vi "Durability_will_2012_07_02_one thing.vi"() -> ()   [LabVIEW 2011]
uses:
  <vilib>/DAQmx/write.llb/DAQmx Write (Counter Time 1Chan 1Samp).vi
  <vilib>/DAQmx/read.llb/DAQmx Read (Analog 1D Wfm NChan NSamp).vi
  <vilib>/DAQmx/create/channels.llb/DAQmx Create Channel (CO-Pulse Generation-Time).vi
  <vilib>/DAQmx/configure/timing.llb/DAQmx Timing (Implicit).vi
  <vilib>/DAQmx/configure/timing.llb/DAQmx Timing (Sample Clock).vi
  <vilib>/DAQmx/create/channels.llb/DAQmx Create Channel (AI-Voltage-Basic).vi
  <vilib>/measure/madcrms.llb/Averaged DC-RMS for 1 Chan.vi
  <vilib>/DAQmx/miscellaneous.llb/DAQmx Fill In Error Info.vi
  <vilib>/measure/NI_MAPro.lvlib
  C:/Program Files/National Instruments/LabVIEW 2011/resource/objmgr/daqmx.rc
panel:
  in  "task in":refnum<k21>
  in  "Physical Channels":tag[](array[tag])
  in  "Channels Name":string[](array[string])
  out "VDE":waveform(dbl)
  out "ICD":waveform(dbl)
  out "VBE":waveform(dbl)
  out "IAB":waveform(dbl)
  out "RPM Graph":dbl(graph)
  out "Motor RPM":dbl format="%#.0f"
  out "Motor Power (watts)":dbl format="%#.4f"
  out "Motor Power Over Time":waveform(dbl)(graph)
  out "Phase to Phase Voltage":waveform(dbl)(graph)
  out "Phase Current":waveform(dbl)(graph)
  out "?":dynamicdata(graph)=[{"t0"=timestamp(3379298263.593967 s since 1904-01-01), "dt"=4.999999999999997e-05, "Y"=array[1000 elements], "attributes"=variant("NI_ChannelName"=variant(string "RPM (Filtered)"), "NI_OriginalChannelName"=variant(string "RPM"), "NI_UnitDescription"=variant(string "Volts"))}]
  in  "Manual Start":bool
  in  "Power \nSetting":i8(slide) min=0 max=100 step=10 scale=0.0..100.0
  in  "Manual Start 2":bool
  out "Boolean 2":bool
  in  "Profile Controls":string[][](table)=[["60", "2", ""], ["70", "4", ""], ["80", "2", ""], ["90", "3", ""], ["100", "3", ""], ["", "", ""], ["", "", ""], ["", "", ""], ["", "", ""], ["", "", ""], ["", "", ""]]
  in  "Quit 4":bool
  out "Power Setting (%)":dbl format="%#.2f"
  out "Boolean":bool
  in  "Power Input":i8
  in  "Run Motor":bool
  # "Motor Power and RPM"
  # "Temperature"
  # "MC1"
  # "RPM"
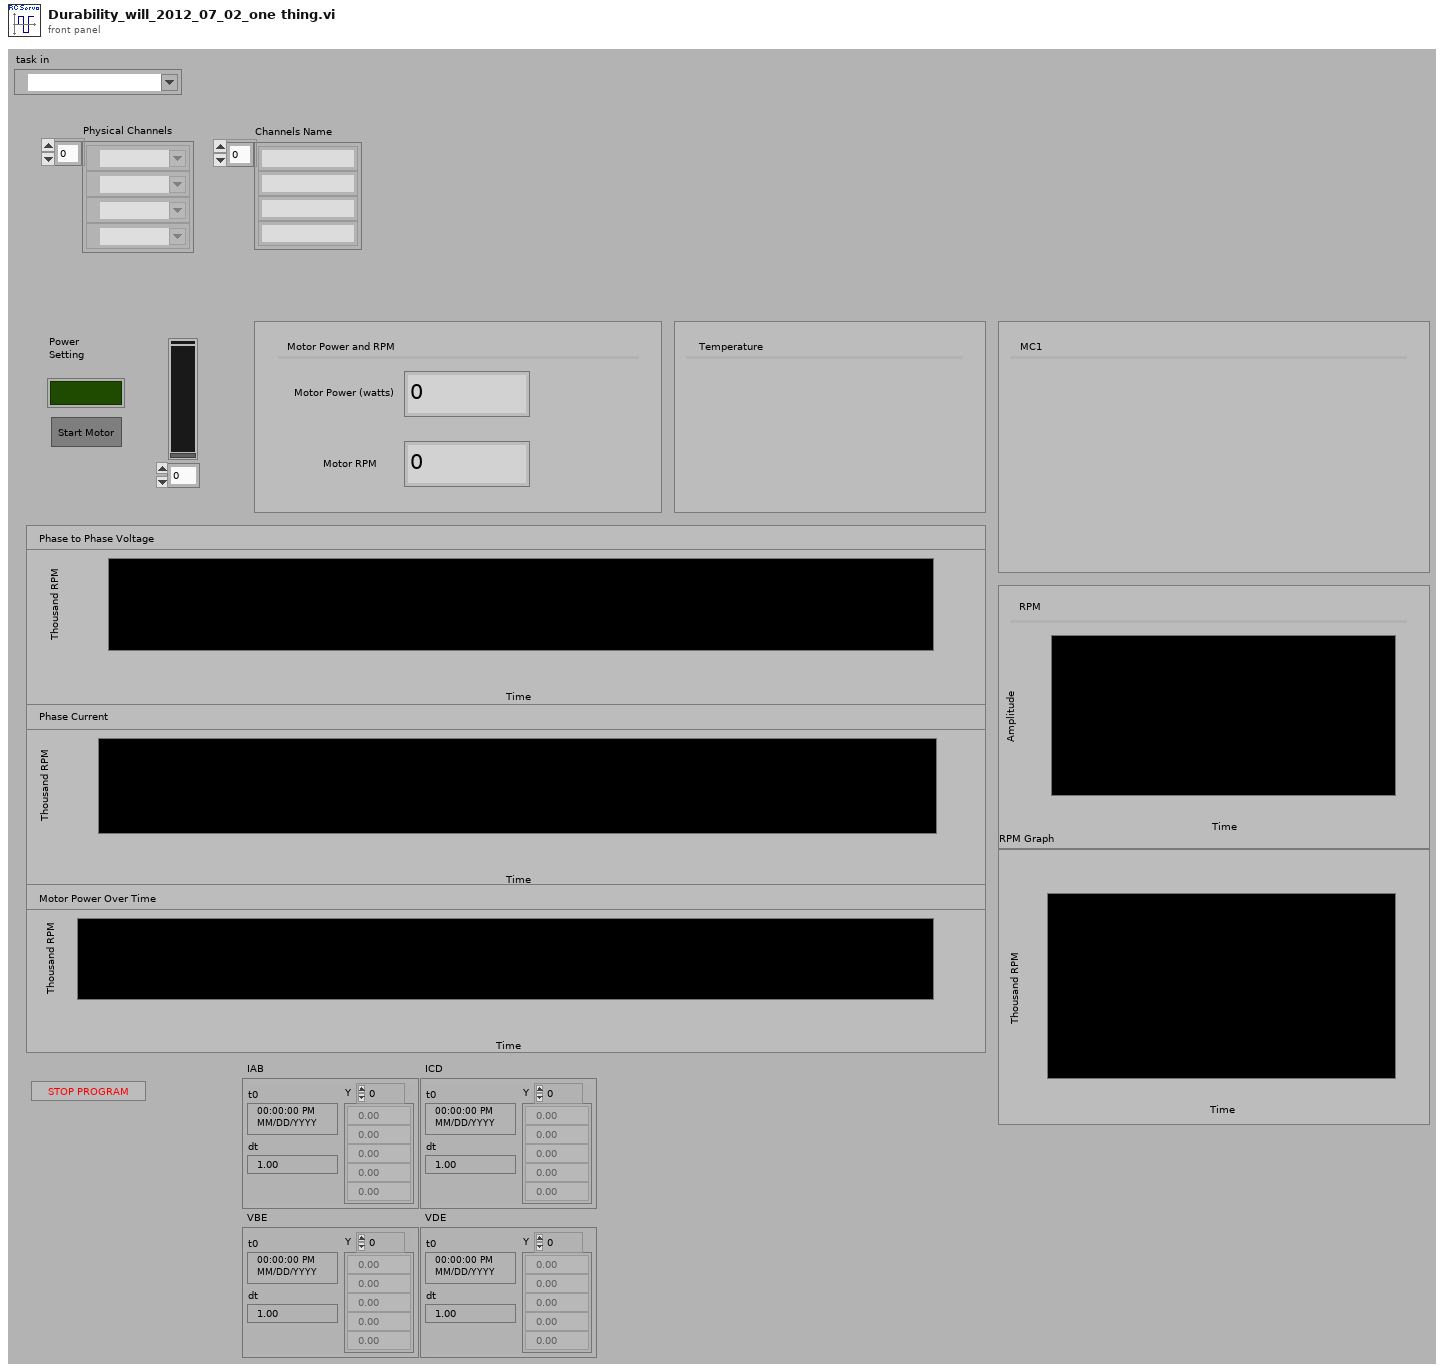
[diagram p1: front panel]
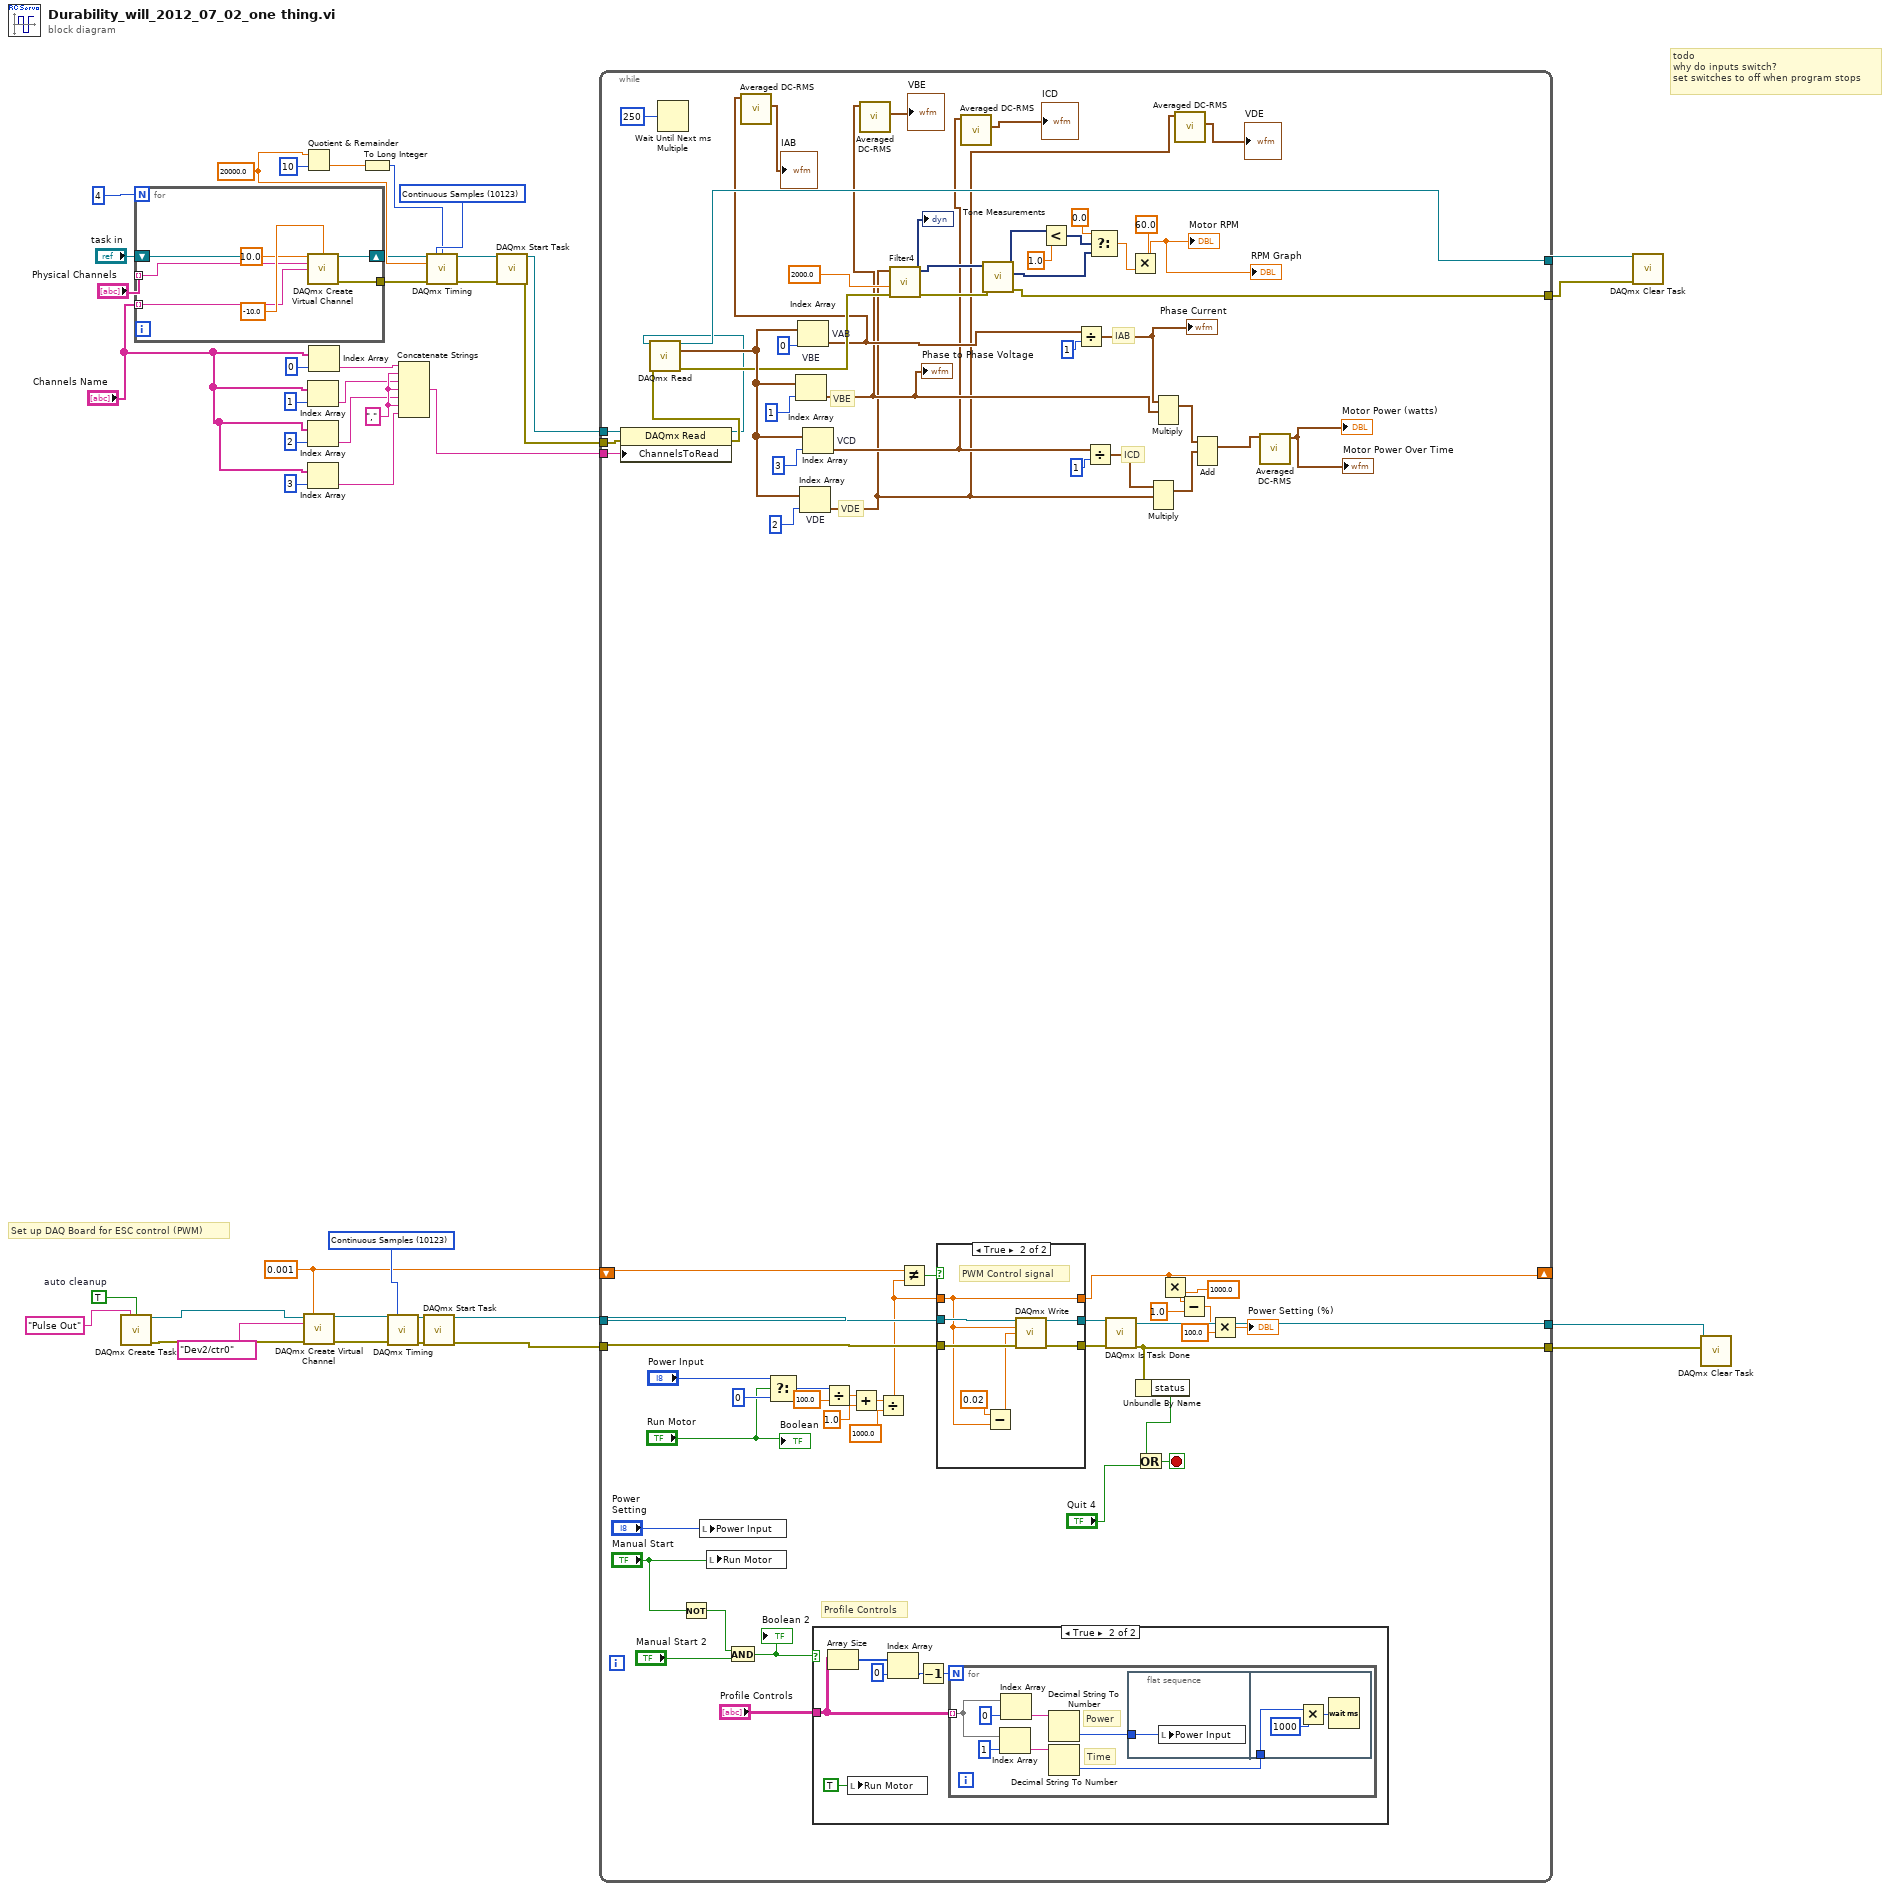
[diagram p0: block diagram]
diagram:
  w7 = "," ("string")
  w20 = 20000.0 ("Sample Rate")
  w25 = 10123 items=["Finite Samples"=10178, "Continuous Samples"=10123] ("sample mode")
  w33 = TRUE  # auto cleanup
  w34 = 0.001 ("y")
  w35 = 10123 items=["Finite Samples"=10178, "Continuous Samples"=10123, "Hardware Timed Single Point"=12522] ("sample mode")
  # "todo\nwhy do inputs switch?\nset switches to off when program stops"
  # "Set up DAQ Board for ESC control (PWM)"
  n1 = call <vilib>:"DAQmx Create Task.vi"("new task name"="Pulse Out", "auto cleanup"=w33) -> ("task out"=w31:refnum<k21>, "error out"=w32:errorcluster)  [unwired: 12 in]
  n2 = for {
    N: 4 -> [_]
    tunnel: "Physical Channels" -> [w46] mode=indexing
    tunnel: "Channels Name" -> [w47] mode=indexing
    tunnel: [w45] -> w17
    shift-right: [w44] -> w15
    shift-left: "task in" -> [w43]
    n3 = call-poly <vilib>:"DAQmx Create Virtual Channel.vi"("task in"=w43, "maximum value"=10.0 ("Maximum Value"), "minimum value"=-10.0 ("Minimum Value"), "physical channels"=w46, "name to assign"=w47) -> ("task out"=w44:refnum<k21>, "error out"=w45:errorcluster)  [unwired: 9 in]
  }
  n4 = Quotient & Remainder(x=w20, y=10 ("samples per channel")) -> (floor(x/y)=w21:dbl)  [unwired: 1 out]
  n5 = call-poly <vilib>:"DAQmx Create Virtual Channel.vi"("task in"=w31, "high time"=w34, "counter"=tag "Dev2/ctr0" ("PWM Output Channel (ctr0)"), "error in"=w32) -> ("task out"=w42:refnum<k21>, "error out"=w41:errorcluster)  [unwired: 10 in]
  n6 = Index Array(array="Channels Name", index=1) -> (element=w5:string)
  n7 = Index Array(array="Channels Name", index=2) -> (element=w3:string)
  n8 = Index Array(array="Channels Name", index=3) -> (element=w4:string)
  n9 = Index Array(array="Channels Name", index=0) -> (element=w6:string)
  n10 = To Long Integer(number=w21) -> (32bit integer=w19:i32)
  n11 = call-poly <vilib>:"DAQmx Timing.vi"("task/channels in"=w42, "sample mode"=w35, "error in"=w41) -> ("task out"=w40:refnum<k21>, "error out"=w39:errorcluster)  [unwired: 11 in]
  n12 = Concatenate Strings(w6, w7, w5, w7, w3, w7, w4) -> (w2:string)
  n13 = call <vilib>:"DAQmx Start Task.vi"("task/channels in"=w40, "error in"=w39) -> ("task out"=w36:refnum<k21>, "error out"=w28:errorcluster)  [unwired: 12 in]
  n14 = call-poly <vilib>:"DAQmx Timing.vi"("task/channels in"=w15, "sample mode"=w25, "samples per channel"=w19, "rate"=w20, "error in"=w17) -> ("task out"=w24:refnum<k21>, "error out"=w23:errorcluster)  [unwired: 9 in]
  n15 = call <vilib>:"DAQmx Start Task.vi"("task/channels in"=w24, "error in"=w23) -> ("task out"=w13:refnum<k21>, "error out"=w12:errorcluster)  [unwired: 12 in]
  n16 = while {
    tunnel: [w124] -> w38
    tunnel: [w123] -> w37
    tunnel: w36 -> [w119]
    tunnel: w28 -> [w118]
    shift-right: [w101] -> _
    shift-left: w34 -> [w109]
    tunnel: [w66] -> w27
    tunnel: [w65] -> w26
    tunnel: w13 -> [w52]
    tunnel: w12 -> [w51]
    tunnel: w2 -> [w50]
    stop <- w122 stop-if-true
    # "IAB"
    # "VBE"
    # "ICD"
    # "VDE"
    # "Profile Controls"
    n17 = property class="DAQmx Read"(reference=w52, error in=w51, "ChannelsToRead"=w50) -> (reference out=w53:refnum<k21>, error out=w54:errorcluster)
    n18 = call-poly <vilib>:"DAQmx Read.vi"("task/channels in"=w53, "error in"=w54) -> ("task out"=w66:refnum<k21>, "data"=w83:waveform(dbl)[], "error out"=w76:errorcluster)  [unwired: 11 in]
    n19 = Wait Until Next ms Multiple(millisecond multiple=u32 250) -> ()  [unwired: 1 out]
    n20 = Not(x="Manual Start") -> (.not. x?=w94:bool)
    n21 = local write "Power Input"("Power \nSetting") -> ()
    n22 = local write "Run Motor"("Manual Start") -> ()
    n23 = And(x=w94, y="Manual Start 2") -> (x .and. y?=w96:bool)
    "Boolean 2" <- w96
    n24 = Select(t="Power Input", s="Run Motor", f=i8 0) -> (s? t:f=w107:i8)
    n25 = Index Array "VBE"(array=w83, index=1) -> (element=w61:waveform(dbl))
    "Phase to Phase Voltage" <- w61
    n26 = Index Array "VAB"(array=w83, index=0) -> (element=w62:waveform(dbl))
    n27 = call-poly <vilib>:"Averaged DC-RMS.vi"("signal in"=w62) -> ("RMS value waveform"=→"IAB":waveform(dbl))  [unwired: 6 in, 4 out]
    n28 = Index Array "VDE"(array=w83, index=2) -> (element=w59:waveform(dbl))
    n29 = Index Array "VCD"(array=w83, index=3) -> (element=w60:waveform(dbl))
    n30 = case shown="True" w96 {
      tunnel: "Profile Controls" -> [_ w126]
      frame False {
      }
      frame True {
        n31 = Array Size(array=w126) -> (size(s)=w130:i32[])
        n32 = local write "Run Motor"(TRUE ("Run Motor")) -> ()
        n33 = Index Array(array=w130, index=0) -> (element=w128:i32)
        n34 = Decrement(x=w128) -> (x-1=w127:i32)
        n35 = for {
          N: w127 -> [_]
          tunnel: w126 -> [w132] mode=indexing
          # "Time"
          # "Power"
          n36 = Index Array(array=w132, index=1) -> (element=w134:string)
          n37 = Index Array(array=w132, index=0) -> (element=w135:string)
          n38 = Decimal String To Number(string=w135) -> (number=w133:i32)  [unwired: 2 in, 1 out]
          n39 = Decimal String To Number(string=w134) -> (number=w131:i32)  [unwired: 2 in, 1 out]
          n40 = flat-sequence {
            tunnel: w133 -> [w138]
            tunnel: w131 -> [w139]
            frame #0 {
              n41 = local write "Power Input"(w138) -> ()
            }
            frame #1 {
              n42 = Multiply(x=w139, y=1000) -> (x*y=w140:i32)
              n43 = Wait (ms)(milliseconds to wait=w140) -> ()  [unwired: 1 out]
            }
          }
        }
      }
    }
    n44 = Divide(x=w107, y=100.0) -> (x/y=w113:dbl)
    n45 = Add(x=w113, y=1.0 ("x/y")) -> (x+y=w111:dbl)
    n46 = call-poly <vilib>:"Averaged DC-RMS.vi"("signal in"=w61) -> ("RMS value waveform"=→"VBE":waveform(dbl))  [unwired: 6 in, 4 out]
    n47 = Divide(x=w111, y=1000.0) -> (x/y=w110:dbl)
    n48 = call "Filter4"("error in (no error)"=w76, "Lower Cut-Off"=2000.0 ("LowPass Filter CutOff [Hz]"), "Signal"=w59) -> ("error out"=w77:errorcluster, "Filtered Signal"=w68:dynamicdata)  [unwired: 7 in]
    "?" <- w68
    n49 = Not Equal?(x=w109, y=w110) -> (x != y?=w120:bool)
    n50 = case shown="True" w120 {
      tunnel: w110 -> [w142 w145]
      tunnel: w119 -> [w144 w150]
      tunnel: w118 -> [w143 w149]
      tunnel: [w144 w147] -> w117
      tunnel: [w143 w146] -> w116
      tunnel: [w142 w145] -> w101
      frame False {
      }
      frame True {
        # "PWM Control signal"
        n51 = Subtract(x=0.02, y=w145) -> (x-y=w148:dbl)
        n52 = call-poly <vilib>:"DAQmx Write.vi"("task/channels in"=w150, "high time"=w145, "low time"=w148, "error in"=w149) -> ("task out"=w147:refnum<k21>, "error out"=w146:errorcluster)  [unwired: 9 in, 1 out]
      }
    }
    n53 = call-poly <vilib>:"Averaged DC-RMS.vi"("signal in"=w60) -> ("RMS value waveform"=→"ICD":waveform(dbl))  [unwired: 6 in, 4 out]
    n54 = call "Tone Measurements"("error in (no error)"=w77, "Signals"=w68) -> ("error out"=w65:errorcluster, "Frequency"=w72:dynamicdata, "Amplitude"=w69:dynamicdata)  [unwired: 7 in]
    n55 = Less?(x=w69, y=1.0) -> (x < y?=w71:dynamicdata)
    n56 = Divide(x=w62, y=1) -> (x/y=w64:waveform(dbl))
    "Phase Current" <- w64
    n57 = Divide(x=w60, y=1) -> (x/y=w87:waveform(dbl))
    n58 = Select(t=0.0, s=w71, f=w72) -> (s? t:f=w74:dbl)
    n59 = call <vilib>:"DAQmx Is Task Done.vi"("task/channels in"=w117, "error in"=w116) -> ("task out"=w124:refnum<k21>, "error out"=w123:errorcluster)  [unwired: 11 in, 1 out]
    n60 = Multiply(x=60.0, y=w74) -> (x*y=→"Motor RPM" →"RPM Graph":dbl)
    n61 = Unbundle By Name(w123) -> ("status"=w121:bool)
    n62 = Or(x=w121, y="Quit 4") -> (x .or. y?=w122:bool)
    n63 = Multiply(1:w59, 2:w87) -> (0:w85:waveform(dbl))  [unwired: 1 in, 1 out]
    n64 = Multiply(1:w61, 2:w64) -> (0:w88:waveform(dbl))  [unwired: 1 in, 1 out]
    n65 = Multiply(x=w101, y=1000.0) -> (x*y=w102:dbl)
    n66 = call-poly <vilib>:"Averaged DC-RMS.vi"("signal in"=w59) -> ("RMS value waveform"=→"VDE":waveform(dbl))  [unwired: 6 in, 4 out]
    n67 = Subtract(x=w102, y=1.0) -> (x-y=w105:dbl)
    n68 = Add(1:w85, 2:w88) -> (0:w89:waveform(dbl))  [unwired: 1 in, 1 out]
    n69 = Multiply(x=w105, y=100.0) -> (x*y=→"Power Setting (%)":dbl)
    n70 = call-poly <vilib>:"Averaged DC-RMS.vi"("signal in"=w89) -> ("DC value waveform"=→"Motor Power Over Time" →"Motor Power (watts)":waveform(dbl))  [unwired: 6 in, 4 out]
    "Boolean" <- "Run Motor"
  }
  n71 = call <vilib>:"DAQmx Clear Task.vi"("task in"=w27, "error in"=w26) -> ()  [unwired: 13 in, 1 out]
  n72 = call <vilib>:"DAQmx Clear Task.vi"("task in"=w38, "error in"=w37) -> ()  [unwired: 13 in, 1 out]
